vi "Initialize.vi"(8 "error in (no error)":errorcluster, 11 "RandomNumberLogger in":refnum<class "RandomNumberLogger.lvclass">) -> (0 "error out":errorcluster, 3 "RandomNumberLogger out":refnum<class "RandomNumberLogger.lvclass">)   [LabVIEW 2020, in "RandomNumberLogger.lvlib" / "RandomNumberLogger.lvclass"]
doc: "<b>Initialize</b>\nThis is called once for the entire lifetime of the plugin, and is where the timing option for the plugin is set if the value is not based on the configuration file.\n\nInitialize is called before the plugin loads its configuration.\n\nTiming options:\n - Periodic: Specify a millisecond period for the Process loop to run at.\n - Immediate: Run the process loop as quickly as possible, with no added delay between calls. Use if the Process loop blocks execution on its own, for instance to wait for DAQ samples to be ready.\n - On Data Ready: Run process whenever data arrives on the Input stream. Use for PEs that process input data.\n - Triggered: Use if you configure triggering on the Input stream to only receive data when a trigger condition applies.\n\nMost plugins will use Immediate if they are the source of data or On Data Ready if they are a sink of data."
uses:
  RandomNumberLogger.lvclass
  RandomNumberLogger.lvclass/RandomNumberLogger.ctl
  <vilib>/FlexLogger/SDK/PluginSDK.lvlibp/PEFClasses/SDK/Processing Element/Processing Element.lvclass
  <vilib>/FlexLogger/SDK/PluginSDK.lvlibp/PEFClasses/SDK/Processing Element/Timing Method.ctl
  <vilib>/FlexLogger/SDK/PluginSDK.lvlibp/PEFClasses/SDK/Processing Element/Timing Parameters.ctl
  <vilib>/ADAS Record/Utilities/ADAS Utilities.lvlib
  C:/Program Files/National Instruments/LabVIEW 2020/vi.lib/FlexLogger/SDK/PluginSDK.lvlibp/PEFClasses/SDK/Processing Element/Processing Element.lvclass
  C:/Projects/GitHub/data-record-ad/IO Plugins/Tutorial Solutions/RandomNumberLogger/PE/RandomNumberLogger.lvclass
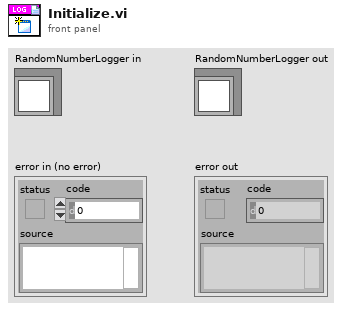
[diagram p1: front panel]
types:
  T1 = typedef "PluginSDK.lvlibp/Processing Element.lvclass/Timing Parameters.ctl" = cluster{"Timing Method":T2, "Timing Period (ms)":i32}
  T2 = typedef "PluginSDK.lvlibp/Processing Element.lvclass/Timing Method.ctl" = enum16{"Periodic", "Immediate", "On Data Ready", "Triggered"}
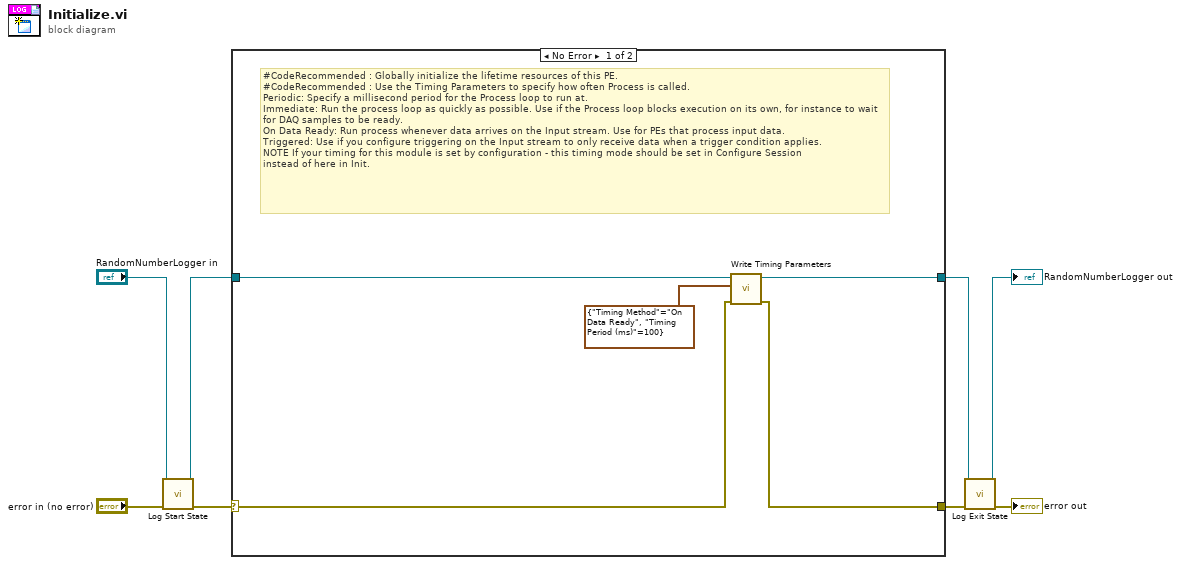
[diagram p0: block diagram]
diagram:
  n1 = call <vilib>:"Log Start State.vi"("error in (no error)"="error in (no error)", "PluginSDK.lvlibp:Processing Element.lvclass"="RandomNumberLogger in") -> ("error out"=w7:errorcluster, "PluginSDK.lvlibp:Processing Element.lvclass"=w5:refnum<class "RandomNumberLogger.lvclass">)  [unwired: 8 in]
  n2 = case shown="No Error" w7 {
    selector: w7 -> [w10 w14]
    tunnel: [w12 w15] -> w2
    tunnel: w5 -> [w13 w15]
    tunnel: [w9 w14] -> w4
    frame No Error {
      # "#CodeRecommended : Globally initialize the lifetime resources of this PE.\n#CodeRecommended : Use the Timing Parameters to specify how often Process is called.\nPeriodic: Specify a millisecond period for the Process loop to run at.\nImmediate: Run the process loop as quickly as possible. Use if the Process loop blocks execution on its own, for instance to wait for DAQ samples to be ready.\nOn Data Ready: Run process whenever data arrives on the Input stream. Use for PEs that process input data.\nTriggered: Use if you configure triggering on the Input stream to only receive data when a trigger condition applies.\nNOTE If your timing for this module is set by configuration - this timing mode should be set in Configure Session\ninstead of here in Init."
      n3 = call <vilib>:"Write Timing Parameters.vi"("error in (no error)"=w10, "Timing Parameters"=T1 {"Timing Method"=enum."On Data Ready", "Timing Period (ms)"=100}, "PEF Processing Element in"=w13) -> ("error out"=w9:errorcluster, "PEF Processing Element out"=w12:refnum<class "RandomNumberLogger.lvclass">)  [unwired: 7 in]
    }
    frame Error {
    }
  }
  n4 = call <vilib>:"Log Exit State.vi"("error in (no error)"=w4, "PluginSDK.lvlibp:Processing Element.lvclass"=w2) -> ("error out"=→"error out":errorcluster, "PluginSDK.lvlibp:Processing Element.lvclass"=→"RandomNumberLogger out":refnum<class "RandomNumberLogger.lvclass">)  [unwired: 8 in]
